vi "Laser349_RS232_Read_Status_List.vi"(8 "error in (no error)":errorcluster, 11 "Laser349 in":refnum<class "Laser349.lvclass">) -> (0 "error out":errorcluster, 1 "Boolean array":bool[](array[boolean]), 2 "Laser_349_status":T1, 3 "Laser349 out":refnum<class "Laser349.lvclass">, 4 "Temperature_Laser_Value":sgl)   [LabVIEW 2018, in "Laser349.lvclass"]
uses:
  Laser349.lvclass
  Ctl/_ctl_LaserStatus.ctl
  Ctl/_ctl_LaserCmd.ctl
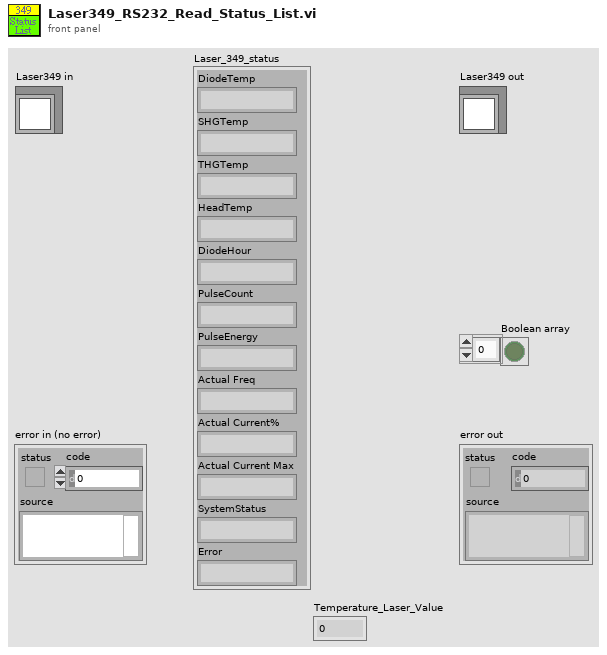
[diagram p1: front panel]
types:
  T1 = typedef "_ctl_LaserStatus.ctl" = cluster{"DiodeTemp":string, "SHGTemp":string, "THGTemp":string, "HeadTemp":string, "DiodeHour":string, "PulseCount":string, "PulseEnergy":string, "Actual Freq":string, "Actual Current%":string, "Actual Current Max":string, "SystemStatus":string, "Error":string}
  T2 = typedef "_ctl_LaserCmd.ctl" = enum8{"Diode_On", "Diode_Off", "Standby_On", "Standby_Off", "Internal_Trig", "External_Trig", "Set_Energy", "Set_Frequency", "Read_Version", "Read_STB", "Read_Diode_TEMP", "Read_SHG_TEMP", "Read_THG_TEMP", "Read_Base_Plate_TEMP", "Read_Diode_Hour", "Read_Diode_Maxc", "Read_Diode_Curr", "Read_QSW_CNTS", "Read_PENER", "Read_Freq", "Read_PCUR", "Read_Fault_Codes"}
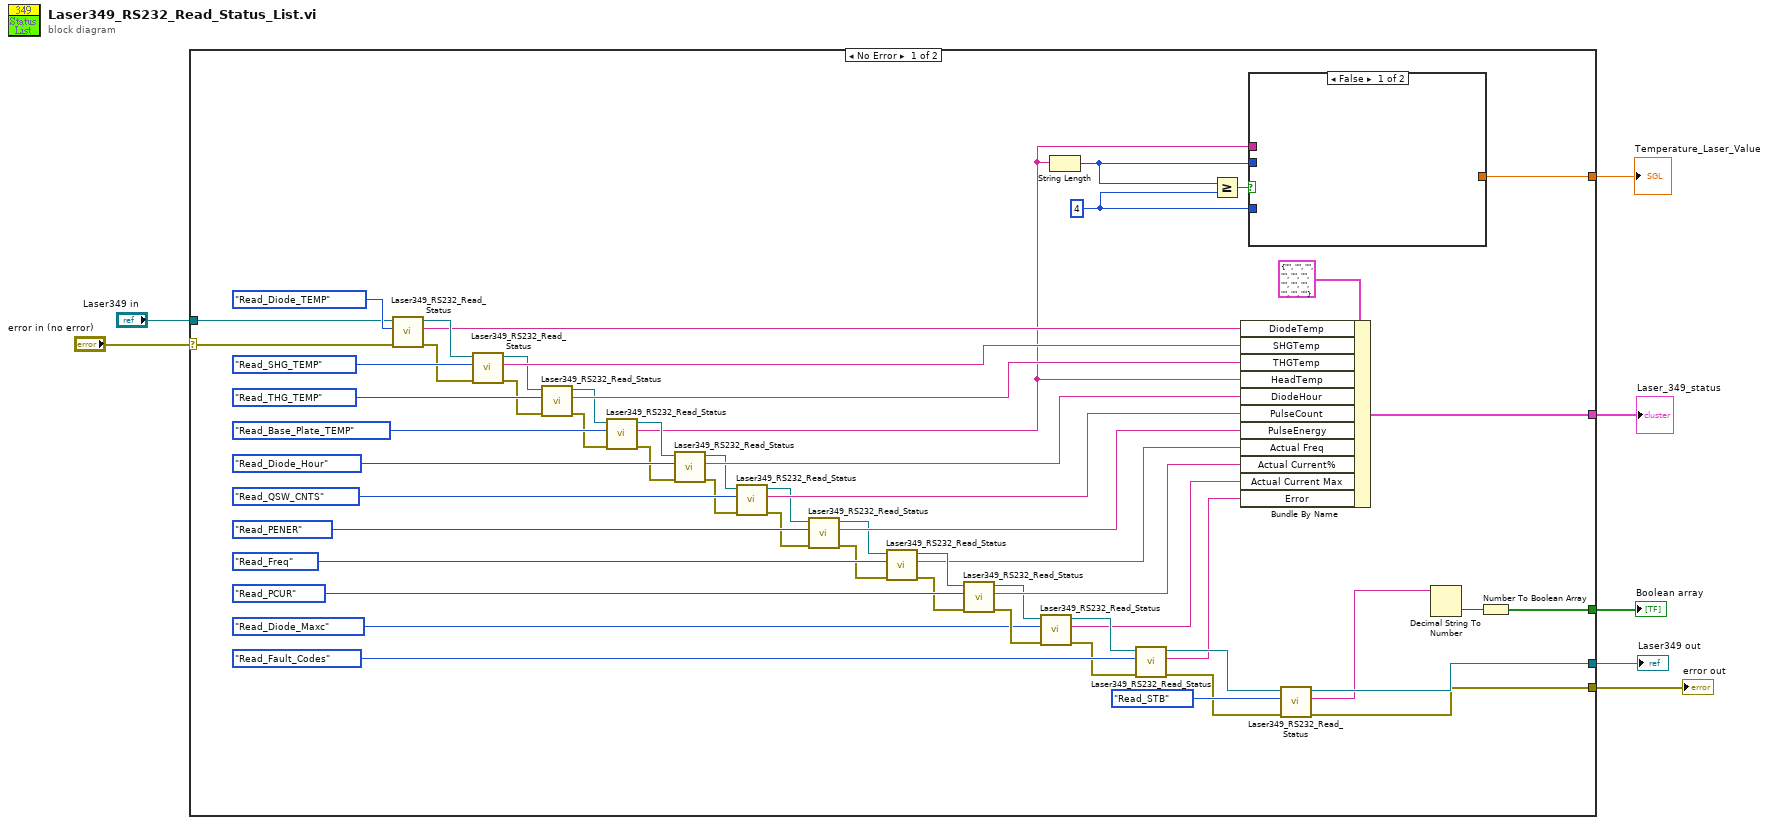
[diagram p0: block diagram]
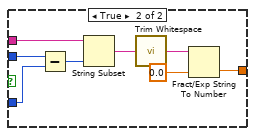
[diagram p2: hidden frame]
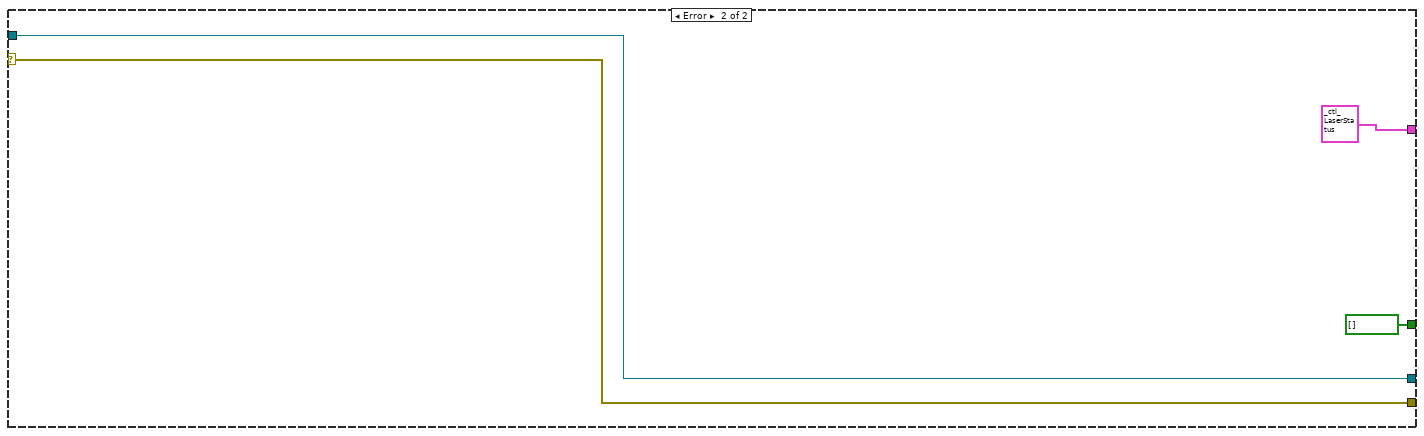
[diagram p3: hidden frame]
diagram:
  n1 = case shown="No Error" "error in (no error)" {
    selector: "error in (no error)" -> [w55 w77]
    tunnel: [w23 w77] -> w6
    tunnel: [w24 w76] -> w4
    tunnel: "Laser349 in" -> [w56 w76]
    tunnel: [w28 T1 {"DiodeTemp"="Error", "SHGTemp"="Error", "THGTemp"="Error", "HeadTemp"="Error", "DiodeHour"="Error", "PulseCount"="Error", "PulseEnergy"="Error", "Actual Freq"="Error", "Actual Current%"="Error", "Actual Current Max"="", "SystemStatus"="", "Error"="Error"} ("Laser_349_status 2")] -> w3
    tunnel: [w18 _] -> w2
    tunnel: [w15 bool[] [] ("Boolean array")] -> w1
    frame No Error {
      w21 = 4 ("y")
      n2 = call-dynamic "Laser349_RS232_Read_Status.vi"("error in (no error)"=w55, "Command Status"=_ctl_LaserCmd."Read_Diode_TEMP", "Laser349 in"=w56) -> ("error out"=w53:errorcluster, "Result String"=w52:string, "Laser349 out"=w54:refnum<class "Laser349.lvclass">)  [unwired: 6 in]
      n3 = call-dynamic "Laser349_RS232_Read_Status.vi"("error in (no error)"=w53, "Command Status"=_ctl_LaserCmd."Read_SHG_TEMP", "Laser349 in"=w54) -> ("error out"=w49:errorcluster, "Result String"=w51:string, "Laser349 out"=w50:refnum<class "Laser349.lvclass">)  [unwired: 6 in]
      n4 = call-dynamic "Laser349_RS232_Read_Status.vi"("error in (no error)"=w49, "Command Status"=_ctl_LaserCmd."Read_THG_TEMP", "Laser349 in"=w50) -> ("error out"=w46:errorcluster, "Result String"=w48:string, "Laser349 out"=w47:refnum<class "Laser349.lvclass">)  [unwired: 6 in]
      n5 = call-dynamic "Laser349_RS232_Read_Status.vi"("error in (no error)"=w46, "Command Status"=_ctl_LaserCmd."Read_Base_Plate_TEMP", "Laser349 in"=w47) -> ("error out"=w45:errorcluster, "Result String"=w19:string, "Laser349 out"=w44:refnum<class "Laser349.lvclass">)  [unwired: 6 in]
      n6 = call-dynamic "Laser349_RS232_Read_Status.vi"("error in (no error)"=w45, "Command Status"=_ctl_LaserCmd."Read_Diode_Hour", "Laser349 in"=w44) -> ("error out"=w42:errorcluster, "Result String"=w43:string, "Laser349 out"=w41:refnum<class "Laser349.lvclass">)  [unwired: 6 in]
      n7 = call-dynamic "Laser349_RS232_Read_Status.vi"("error in (no error)"=w42, "Command Status"=_ctl_LaserCmd."Read_QSW_CNTS", "Laser349 in"=w41) -> ("error out"=w32:errorcluster, "Result String"=w38:string, "Laser349 out"=w33:refnum<class "Laser349.lvclass">)  [unwired: 6 in]
      n8 = call-dynamic "Laser349_RS232_Read_Status.vi"("error in (no error)"=w32, "Command Status"=_ctl_LaserCmd."Read_PENER", "Laser349 in"=w33) -> ("error out"=w30:errorcluster, "Result String"=w36:string, "Laser349 out"=w31:refnum<class "Laser349.lvclass">)  [unwired: 6 in]
      n9 = call-dynamic "Laser349_RS232_Read_Status.vi"("error in (no error)"=w30, "Command Status"=_ctl_LaserCmd."Read_Freq", "Laser349 in"=w31) -> ("error out"=w39:errorcluster, "Result String"=w35:string, "Laser349 out"=w40:refnum<class "Laser349.lvclass">)  [unwired: 6 in]
      n10 = call-dynamic "Laser349_RS232_Read_Status.vi"("error in (no error)"=w39, "Command Status"=_ctl_LaserCmd."Read_PCUR", "Laser349 in"=w40) -> ("error out"=w12:errorcluster, "Result String"=w34:string, "Laser349 out"=w14:refnum<class "Laser349.lvclass">)  [unwired: 6 in]
      n11 = call-dynamic "Laser349_RS232_Read_Status.vi"("error in (no error)"=w12, "Command Status"=_ctl_LaserCmd."Read_Diode_Maxc", "Laser349 in"=w14) -> ("error out"=w11:errorcluster, "Result String"=w8:string, "Laser349 out"=w13:refnum<class "Laser349.lvclass">)  [unwired: 6 in]
      n12 = String Length(string=w19) -> (length=w22:i32)
      n13 = call-dynamic "Laser349_RS232_Read_Status.vi"("error in (no error)"=w11, "Command Status"=_ctl_LaserCmd."Read_Fault_Codes", "Laser349 in"=w13) -> ("error out"=w25:errorcluster, "Result String"=w9:string, "Laser349 out"=w26:refnum<class "Laser349.lvclass">)  [unwired: 6 in]
      n14 = Greater Or Equal?(x=w22, y=w21) -> (x >= y?=w20:bool)
      n15 = Bundle By Name(cluster=T1 {"DiodeTemp"="", "SHGTemp"="", "THGTemp"="", "HeadTemp"="", "DiodeHour"="", "PulseCount"="", "PulseEnergy"="", "Actual Freq"="", "Actual Current%"="", "Actual Current Max"="", "SystemStatus"="", "Error"=""} ("Laser_349_status 2"), "DiodeTemp"=w52, "SHGTemp"=w51, "THGTemp"=w48, "HeadTemp"=w19, "DiodeHour"=w43, "PulseCount"=w38, "PulseEnergy"=w36, "Actual Freq"=w35, "Actual Current%"=w34, "Actual Current Max"=w8, "Error"=w9) -> (w28:T1)
      n16 = case shown="False" w20 {
        tunnel: w22 -> [_ w73]
        tunnel: w21 -> [_ w72]
        tunnel: w19 -> [_ w70]
        tunnel: [_ w66] -> w18
        frame False {
        }
        frame True {
          n17 = Subtract(x=w73, y=w72) -> (x-y=w71:i32)
          n18 = String Subset(string=w70, length (rest)=w71) -> (substring=w69:string)  [unwired: 1 in]
          n19 = call <vilib>:"Trim Whitespace.vi"("string"=w69) -> ("trimmed string"=w68:string)  [unwired: 1 in]
          n20 = Fract/Exp String To Number(string=w68, default (0 dbl)=sgl 0.0 ("default (0 DBL)")) -> (number=w66:sgl)  [unwired: 2 in, 1 out]
        }
      }
      n21 = call-dynamic "Laser349_RS232_Read_Status.vi"("error in (no error)"=w25, "Command Status"=_ctl_LaserCmd."Read_STB", "Laser349 in"=w26) -> ("error out"=w23:errorcluster, "Result String"=w16:string, "Laser349 out"=w24:refnum<class "Laser349.lvclass">)  [unwired: 6 in]
      n22 = Decimal String To Number(string=w16) -> (number=w17:i32)  [unwired: 2 in, 1 out]
      n23 = Number To Boolean Array(number=w17) -> (Boolean array=w15:bool[])
    }
    frame Error {
    }
  }
  "error out" <- w6
  "Laser349 out" <- w4
  "Laser_349_status" <- w3
  "Temperature_Laser_Value" <- w2
  "Boolean array" <- w1
